vi "WRITE Falcon500 values.vi"(0 "PhoenixMotorControlDevRef":T1, 1 "refnum name":string, 3 "error in (no error)":errorcluster) -> (6 "PhoenixMotorControlDevRef 2":T1={"DeviceStatus"={"status"=FALSE, "code"=0, "source"=""}, "Type"=enum."PWM", "PWM"={"PWM Channel"=enum."Invalid", "DeadBand"={"Name"="", "maxPositivePwm"=0, "minPositivePwm"=0, "centerPwm"=0, "maxNegativePwm"=0, "minNegativePwm"=0, "angularRange"=0}}, "CAN"={"Device Number"=0, "SetOutput VI Ref"=variant(enum8{"Percent VBus", "Current", "Speed", "Position", "Voltage"} enum."Percent VBus"), "GetOutput VI Ref"=variant(refnum<k1> refnum), "Enable VI Ref"=variant(dbl 12.0), "Disable VI Ref"=variant(enum8{"Percent VBus", "Speed", "Position", "Slave", "Unchanged / Invalid", "Voltage Compensation", "Current", "Motion Profile"} enum."Percent VBus"), "Data"=variant}, "Invert"=FALSE, "DIO PWM"={"PWM \"Enable\" Channel"=enum."Invalid", "DIOChannel"=enum."Invalid", "PWM Rate"=0.0}}, 9 "error out":errorcluster)   [LabVIEW 2020]
uses:
  <vilib>/Rock Robotics/WPI/MotorControl/WPI_MotorControlDeviceRef.ctl
  <vilib>/Rock Robotics/WPI/MotorControl/WPI_MotorControlType.ctl
  <vilib>/Rock Robotics/SystemInterfaces/DIO/FPGA_DIOPWMChannel.ctl
  <vilib>/Rock Robotics/WPI/PWM/WPI_PWMDeadband.ctl
  <vilib>/Rock Robotics/SystemInterfaces/DIO/FPGA_DIOChannel.ctl
  <vilib>/Rock Robotics/WPI/ThirdParty/Phoenix-LabVIEW/Motor Controller/Get/CTRE_Phoenix_MotorController_IntegratedSensorData_TalonFX.vi
  <vilib>/Rock Robotics/Network Tables/NT Write Number.vi
  <vilib>/Rock Robotics/WPI/ThirdParty/Phoenix-LabVIEW/Motor Controller/Get/CTRE_Phoenix_MotorController_GetTemperature.vi
  <vilib>/Rock Robotics/WPI/ThirdParty/Phoenix-LabVIEW/Motor Controller/Get/CTRE_Phoenix_MotorController_GetSelectedSensorData.vi
  <vilib>/Rock Robotics/WPI/ThirdParty/Phoenix-LabVIEW/Motor Controller/Get/CTRE_Phoenix_MotorController_GetLimitSwitchStates.vi
  <vilib>/Rock Robotics/Network Tables/NT Write Boolean.vi
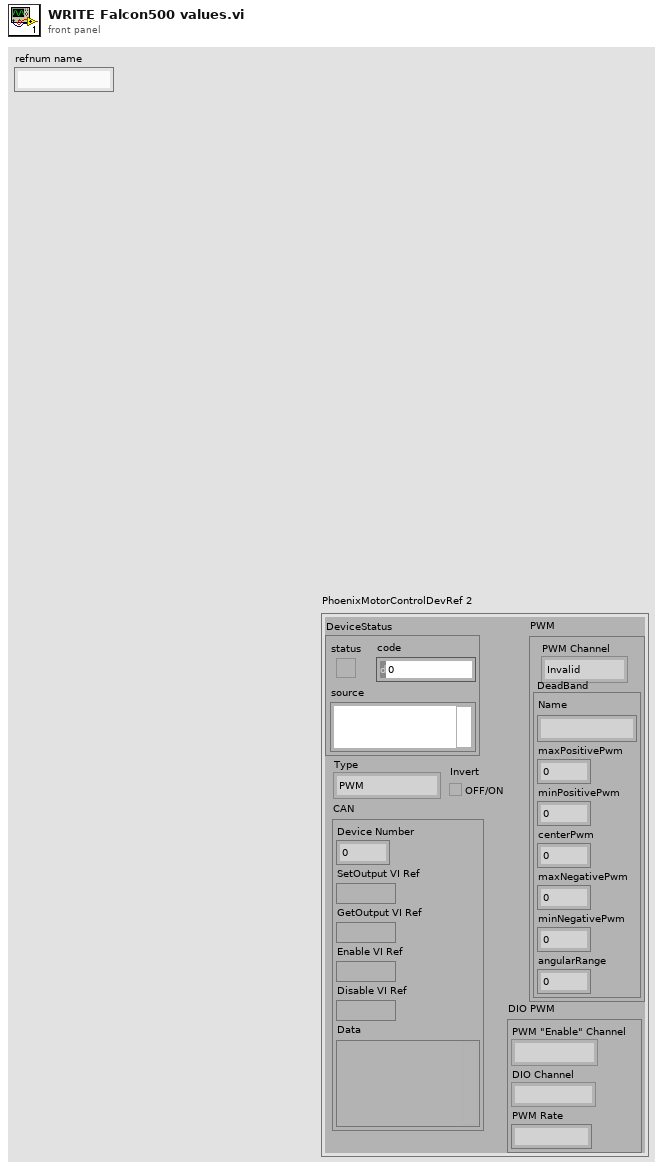
[diagram p1: front panel]
types:
  T1 = typedef "WPI_MotorControlDeviceRef.ctl" = cluster{"DeviceStatus":errorcluster, "Type":T2, "PWM":cluster{"PWM Channel":T3, "DeadBand":T4}, "CAN":cluster{"Device Number":u8, "SetOutput VI Ref":variant, "GetOutput VI Ref":variant, "Enable VI Ref":variant, "Disable VI Ref":variant, "Data":variant}, "Invert":bool, "DIO PWM":cluster{"PWM \"Enable\" Channel":T3, "DIOChannel":T5, "PWM Rate":dbl}}
  T2 = typedef "WPI_MotorControlType.ctl" = enum16{"PWM", "CAN", "DIO PWM"}
  T3 = typedef "FPGA_DIOPWMChannel.ctl" = enum8{"PWM 0", "PWM 1", "PWM 2", "PWM 3", "PWM 4", "PWM 5", "PWM 6", "PWM 7", "PWM 8", "PWM 9", "PWM MXP 0", "PWM MXP 1", "PWM MXP 2", "PWM MXP 3", "PWM MXP 4", "PWM MXP 5", "PWM MXP 6", "PWM MXP 7", "PWM MXP 8", "PWM MXP 9", "Invalid"}
  T4 = typedef "WPI_PWMDeadband.ctl" = cluster{"Name":string, "maxPositivePwm":i32, "minPositivePwm":i32, "centerPwm":i32, "maxNegativePwm":i32, "minNegativePwm":i32, "angularRange":u16}
  T5 = typedef "FPGA_DIOChannel.ctl" = enum8{"DIO 0", "DIO 1", "DIO 2", "DIO 3", "DIO 4", "DIO 5", "DIO 6", "DIO 7", "DIO 8", "DIO 9", "DIO MXP 0", "DIO MXP 1", "DIO MXP 2", "DIO MXP 3", "DIO MXP 4", "DIO MXP 5", "DIO MXP 6", "DIO MXP 7", "DIO MXP 8", "DIO MXP 9", "DIO MXP 10", "DIO MXP 11", "DIO MXP 12", "DIO MXP 13", "DIO MXP 14", "DIO MXP 15", "SPI Port CS1", "SPI Port CS2", "SPI Port CS3", "SPI Port MISO", "SPI Port MOSI", "Invalid"}
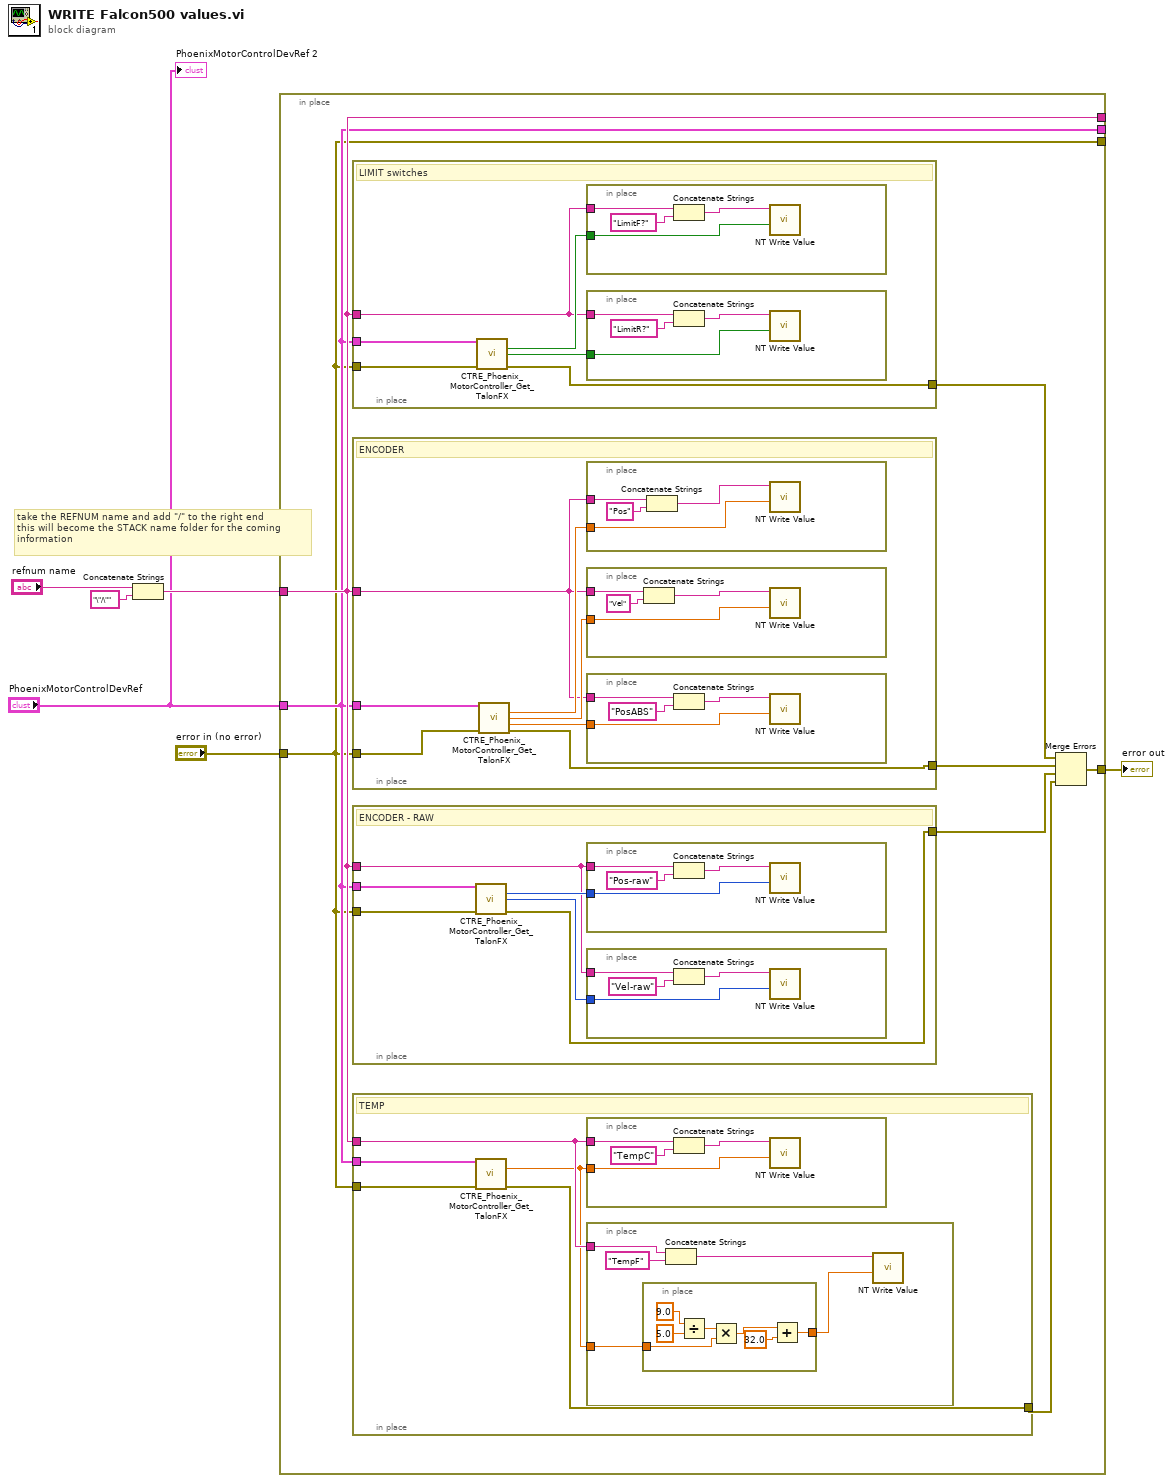
[diagram p0: block diagram]
diagram:
  # "take the REFNUM name and add \"/\" to the right end\nthis will become the STACK name folder for the coming\ninformation"
  n1 = Concatenate Strings("refnum name", "\"/\"" ("string")) -> (w3:string)
  n2 = in-place {
    in-place-border: "PhoenixMotorControlDevRef" -> [w9]
    in-place-border: "error in (no error)" -> [w8]
    in-place-border: w3 -> [w10]
    in-place-border: [w14] -> w1
    in-place-border: [w8] -> _
    in-place-border: [w9] -> _
    in-place-border: [w10] -> _
    n3 = in-place {
      in-place-border: w9 -> [w74]
      in-place-border: w8 -> [w73]
      in-place-border: [w70] -> w12
      in-place-border: w10 -> [w69]
      # "LIMIT switches"
      n4 = call-poly <vilib>:"CTRE_Phoenix_MotorController_Get_TalonFX.vi"("PhoenixMotorControlDevRef"=w74, "error in"=w73) -> ("Forward Limit Closed?"=w72:bool, "Reverse Limit Closed?"=w71:bool, "error out"=w70:errorcluster)  [unwired: 10 in, 1 out]
      n5 = in-place {
        in-place-border: w72 -> [w82]
        in-place-border: w69 -> [w81]
        n6 = Concatenate Strings(w81, "LimitF?" ("string")) -> (w80:string)
        n7 = call-poly <vilib>:"NT Write Value.vi"("Boolean"=w82, "Name"=w80) -> ()  [unwired: 9 in, 1 out]
      }
      n8 = in-place {
        in-place-border: w71 -> [w78]
        in-place-border: w69 -> [w77]
        n9 = Concatenate Strings(w77, "LimitR?" ("string")) -> (w76:string)
        n10 = call-poly <vilib>:"NT Write Value.vi"("Boolean"=w78, "Name"=w76) -> ()  [unwired: 9 in, 1 out]
      }
    }
    n11 = in-place {
      in-place-border: w9 -> [w56]
      in-place-border: [w52] -> w13
      in-place-border: w8 -> [w51]
      in-place-border: w10 -> [w50]
      # "ENCODER"
      n12 = call-poly <vilib>:"CTRE_Phoenix_MotorController_Get_TalonFX.vi"("PhoenixMotorControlDevRef"=w56, "error in"=w51) -> ("Position"=w55:dbl, "Velocity"=w54:dbl, "Absolute Position"=w53:dbl, "error out"=w52:errorcluster)  [unwired: 9 in, 1 out]
      n13 = in-place {
        in-place-border: w55 -> [w66]
        in-place-border: w50 -> [w65]
        n14 = Concatenate Strings(w65, "Pos" ("string")) -> (w68:string)
        n15 = call-poly <vilib>:"NT Write Value.vi"("Numeric"=w66, "Name"=w68) -> ()  [unwired: 9 in, 1 out]
      }
      n16 = in-place {
        in-place-border: w54 -> [w62]
        in-place-border: w50 -> [w61]
        n17 = Concatenate Strings(w61, "Vel" ("string")) -> (w64:string)
        n18 = call-poly <vilib>:"NT Write Value.vi"("Numeric"=w62, "Name"=w64) -> ()  [unwired: 9 in, 1 out]
      }
      n19 = in-place {
        in-place-border: w53 -> [w58]
        in-place-border: w50 -> [w57]
        n20 = Concatenate Strings(w57, "PosABS" ("string")) -> (w60:string)
        n21 = call-poly <vilib>:"NT Write Value.vi"("Numeric"=w58, "Name"=w60) -> ()  [unwired: 9 in, 1 out]
      }
    }
    n22 = in-place {
      in-place-border: w9 -> [w41]
      in-place-border: [w38] -> w11
      in-place-border: w8 -> [w37]
      in-place-border: w10 -> [w36]
      # "ENCODER - RAW"
      n23 = call-poly <vilib>:"CTRE_Phoenix_MotorController_Get_TalonFX.vi"("PhoenixMotorControlDevRef"=w41, "error in"=w37) -> ("Position (Raw Sensor Units)"=w40:i32, "Velocity (Raw Sensor Units per 100 ms)"=w39:i32, "error out"=w38:errorcluster)  [unwired: 10 in, 1 out]
      n24 = in-place {
        in-place-border: w40 -> [w47]
        in-place-border: w36 -> [w46]
        n25 = Concatenate Strings(w46, "Pos-raw" ("string")) -> (w49:string)
        n26 = call-poly <vilib>:"NT Write Value.vi"("Numeric"=w47, "Name"=w49) -> ()  [unwired: 9 in, 1 out]
      }
      n27 = in-place {
        in-place-border: w39 -> [w43]
        in-place-border: w36 -> [w42]
        n28 = Concatenate Strings(w42, "Vel-raw" ("string")) -> (w45:string)
        n29 = call-poly <vilib>:"NT Write Value.vi"("Numeric"=w43, "Name"=w45) -> ()  [unwired: 9 in, 1 out]
      }
    }
    n30 = in-place {
      in-place-border: w9 -> [w19]
      in-place-border: [w18] -> w7
      in-place-border: w8 -> [w17]
      in-place-border: w10 -> [w16]
      # "TEMP"
      n31 = call-poly <vilib>:"CTRE_Phoenix_MotorController_Get_TalonFX.vi"("PhoenixMotorControlDevRef"=w19, "error in"=w17) -> ("Temperature (C)"=w15:dbl, "error out"=w18:errorcluster)  [unwired: 11 in, 1 out]
      n32 = in-place {
        in-place-border: w15 -> [w33]
        in-place-border: w16 -> [w32]
        n33 = Concatenate Strings(w32, "TempC" ("string")) -> (w35:string)
        n34 = call-poly <vilib>:"NT Write Value.vi"("Numeric"=w33, "Name"=w35) -> ()  [unwired: 9 in, 1 out]
      }
      n35 = in-place {
        in-place-border: w16 -> [w22]
        in-place-border: w15 -> [w21]
        n36 = in-place {
          in-place-border: w21 -> [w31]
          in-place-border: [w28] -> w20
          n37 = Divide(x=9.0, y=5.0) -> (x/y=w26:dbl)
          n38 = Multiply(x=w26, y=w31) -> (x*y=w29:dbl)
          n39 = Add(x=w29, y=32.0) -> (x+y=w28:dbl)
        }
        n40 = Concatenate Strings(w22, "TempF" ("string")) -> (w24:string)
        n41 = call-poly <vilib>:"NT Write Value.vi"("Numeric"=w20, "Name"=w24) -> ()  [unwired: 9 in, 1 out]
      }
    }
    n42 = Merge Errors(w12, w13, w11, w7) -> (w14:errorcluster)
  }
  "error out" <- w1
  "PhoenixMotorControlDevRef 2" <- "PhoenixMotorControlDevRef"
